vi "go.vi"(5 "dispense":T3={"Vacuum Setting (0000)"=0, "Pressure"=20, "on delay (ms)"=0.5, "off delay (ms) "=0.5} {"Vacuum Setting (0000)" min=0 max=1000 step=1 format="%04.0f"}, 7 "motion":T2, 8 "use new/data":bool, 9 "file path (dialog if empty)":path=path "D:/Gantry_General/Main/ms_kao/data/CAD PCB full 0.8 P30 20210608/CAD PCB full 0.8 P30 20210608.txt", 10 "cluster Array input":T5(array[cluster]), 11 "controller in":T4) -> (3 "controller out":T4)   [LabVIEW 2016]
uses:
  Classes/Controller/Motion/A3200 Folder/A3200.lvclass
  D:/Gantry_General/Classes/Controller/Motion/Motion Folder/Motion.lvclass
  Classes/Controller/Dispenser/Ultimus V2 Folder/Ultimus V2.lvclass
  Classes/Controller/I-O/NI-DAQ Folder/NI-DAQ.lvclass
  Classes/Controller/Motion/Motion Folder/Motion.lvclass
  Classes/Controller/I-O/I-O Folder/I-O.lvclass
  Classes/Controller/Dispenser/Dispenser Folder/Dispenser.lvclass
  <vilib>/Utility/file.llb/Read Delimited Spreadsheet (DBL).vi
  <vilib>/Utility/file.llb/Write Delimited Spreadsheet (I64).vi
panel:
  out "element":dbl
  out "all rows":dbl[][](array[numeric])
  out "draw point Cluster":T1
  out "Numeric":dbl=0.237
  out "i":i32=23
  out "size(s)":i32=75
  # "使用新/資料"
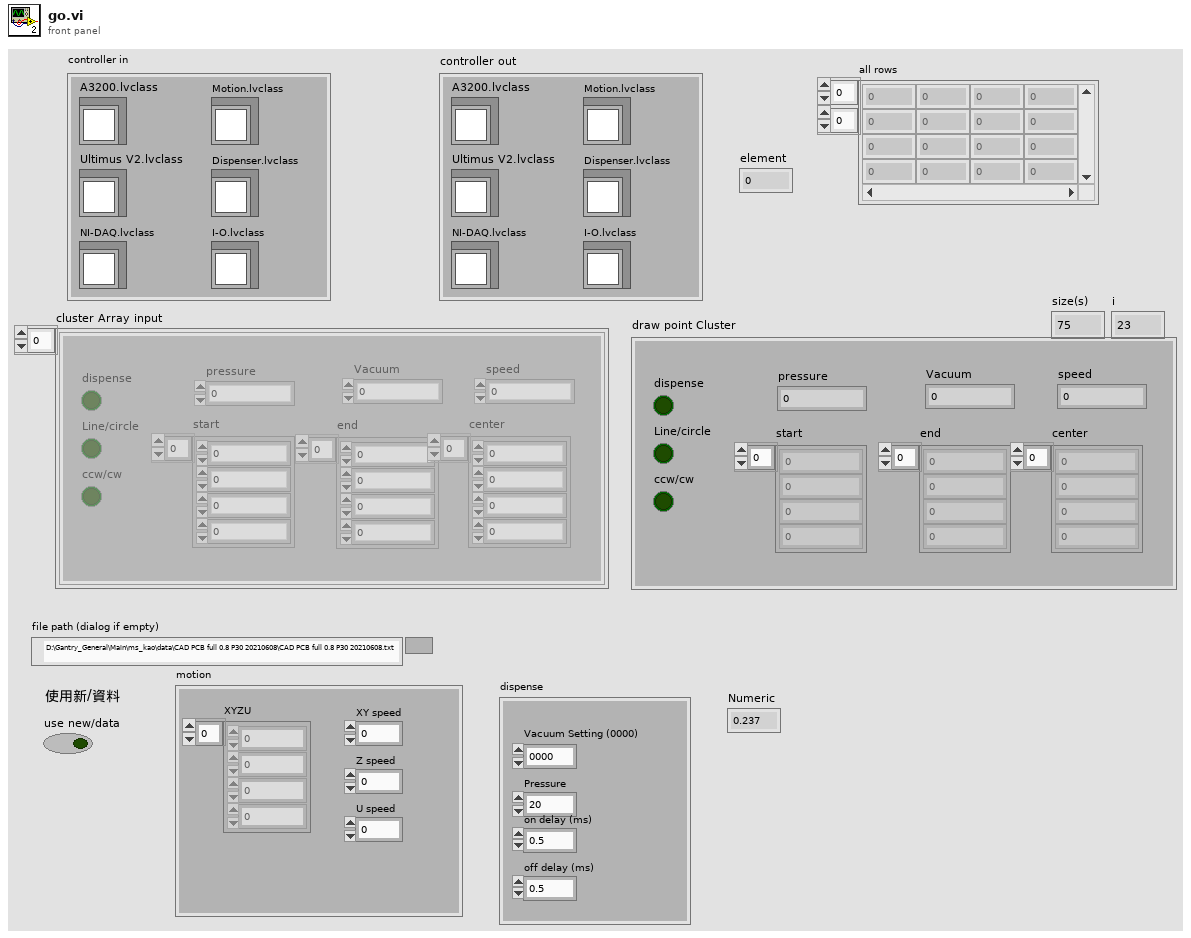
[diagram p1: front panel]
types:
  T1 = cluster{"dispense":bool, "Line/circle":bool, "ccw/cw":bool, "pressure":dbl, "speed":dbl, "start":dbl[], "end":dbl[], "center":dbl[], "Vacuum":dbl}
  T2 = cluster{"XYZU ":dbl[], "XY speed":dbl, "Z speed":dbl, "U speed":dbl}
  T3 = cluster{"Vacuum Setting (0000)":i64, "Pressure":i16, "on delay (ms)":dbl, "off delay (ms) ":dbl}
  T4 = cluster{"A3200.lvclass":refnum<class "A3200.lvclass">, "Ultimus V2.lvclass":refnum<class "Ultimus V2.lvclass">, "NI-DAQ.lvclass":refnum<class "NI-DAQ.lvclass">, "Motion.lvclass":refnum<class "Motion.lvclass">, "I-O.lvclass":refnum<class "I-O.lvclass">, "Dispenser.lvclass":refnum<class "Dispenser.lvclass">}
  T5 = cluster{"dispense":bool, "Line/circle":bool, "ccw/cw":bool, "pressure":dbl, "speed":dbl, "start":dbl[], "end":dbl[], "center":dbl[], "Vacuum":dbl}[]
  T6 = cluster{"file exists":bool, "dispense status now(on)":bool, "dispense status next(off)":bool, "dispense status IN":bool, "dispense status last":bool}
  T7 = typedef "dispense status data.ctl" = cluster{"file exists":bool, "dispense status now(on)":bool, "dispense status next(off)":bool, "dispense status IN":bool, "dispense status last":bool}
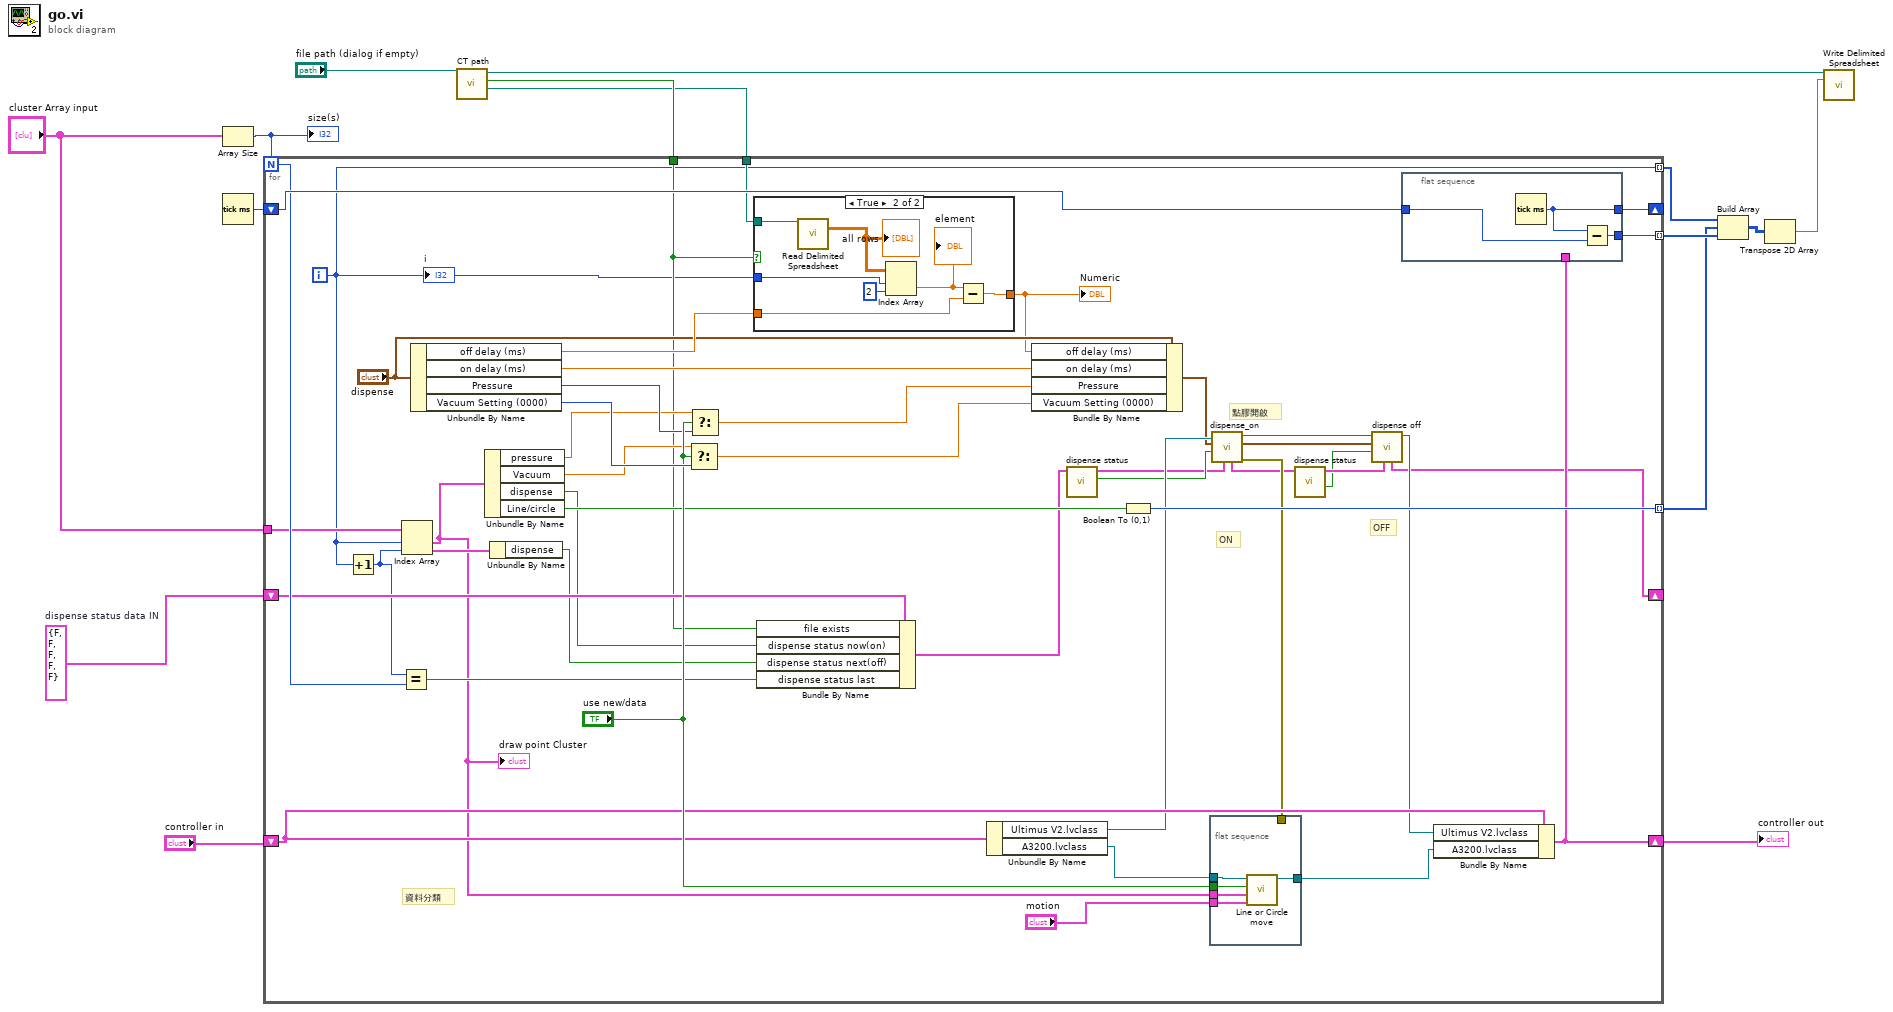
[diagram p0: block diagram]
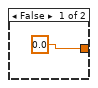
[diagram p2: hidden frame]
diagram:
  w1 = T6 {"file exists"=FALSE, "dispense status now(on)"=FALSE, "dispense status next(off)"=FALSE, "dispense status IN"=FALSE, "dispense status last"=FALSE}  # dispense status data IN
  n1 = Array Size(array="cluster Array input") -> (size(s)=w12:i32)
  "size(s)" <- w12
  n2 = Tick Count (ms)() -> (millisecond timer value=w11:u32)
  n3 = call "CT path.vi"("path"="file path (dialog if empty)") -> ("path 1"=w2:path, "file exists?"=w8:bool, "path 2"=w3:path)  [unwired: 8 in]
  n4 = for {
    N: w12 -> [w51]
    shift-right: [w60] -> _
    shift-left: w11 -> [w61]
    tunnel: [w59] -> w15 mode=indexing
    tunnel: [w58] -> w13 mode=indexing
    tunnel: "cluster Array input" -> [w28]
    tunnel: w8 -> [w29]
    tunnel: w2 -> [w57]
    tunnel: [w20] -> w6 mode=indexing
    shift-right: [w46] -> w4
    shift-left: "controller in" -> [w48]
    shift-right: [w24] -> _
    shift-left: w1 -> [w31]
    i -> [w20]
    # "OFF"
    # "ON"
    # "點膠開啟"
    # "資料分類"
    n5 = Increment(x=w20) -> (x+1=w27:i32)
    n6 = Equal?(x=w27, y=w51) -> (x = y?=w23:bool)
    n7 = Index Array(array=w28, index #1=w20, index #2=w27) -> (element #1=w16:T1, element #2=w26:T1)
    "draw point Cluster" <- w16
    n8 = Unbundle By Name("dispense") -> ("off delay (ms)"=w55:dbl, "on delay (ms)"=w41:dbl, "Pressure"=w49:i16, "Vacuum Setting (0000)"=w56:i64)
    n9 = Unbundle By Name(w16) -> ("pressure"=w37:dbl, "Vacuum"=w36:dbl, "dispense"=w21:bool, "Line/circle"=w50:bool)
    n10 = Unbundle By Name(w26) -> ("dispense"=w22:bool)
    n11 = Select(t=w36, s="use new/data", f=w56) -> (s? t:f=w38:dbl)
    n12 = Select(t=w37, s="use new/data", f=w49) -> (s? t:f=w39:dbl)
    n13 = case shown="True" w29 {
      tunnel: w57 -> [_ w74]
      tunnel: [0.0 ("f") w70] -> w40
      tunnel: w20 -> [_ w69]
      tunnel: w55 -> [_ w68]
      frame False {
      }
      frame True {
        n14 = call-poly <vilib>:"Read Delimited Spreadsheet.vi"("file path (dialog if empty)"=w74) -> ("all rows"=w72:dbl[][])  [unwired: 9 in, 5 out]
        "all rows" <- w72
        n15 = Index Array(array=w72, index (row)=w69, index (col)=2 ("disabled index (col)")) -> (element=w73:dbl)
        "element" <- w73
        n16 = Subtract(x=w73, y=w68) -> (x-y=w70:dbl)
      }
    }
    "Numeric" <- w40
    n17 = Bundle By Name(cluster=w31, "file exists"=w29, "dispense status now(on)"=w21, "dispense status next(off)"=w22, "dispense status last"=w23) -> (w30:T7)
    n18 = Unbundle By Name(w48) -> ("Ultimus V2.lvclass"=w45:refnum<class "Ultimus V2.lvclass">, "A3200.lvclass"=w52:refnum<class "A3200.lvclass">)
    n19 = Bundle By Name(cluster="dispense", "off delay (ms)"=w40, "on delay (ms)"=w41, "Pressure"=w39, "Vacuum Setting (0000)"=w38) -> (w43:T3)
    n20 = call "dispense status.vi"("dispense status data IN"=w30) -> ("dispense run on"=w32:bool, "dispense status data OUT"=w25:T7)  [unwired: 8 in, 1 out]
    n21 = Boolean To (0,1)(Boolean=w50) -> (0, 1=w58:i16)
    n22 = flat-sequence {
      tunnel: "use new/data" -> [w66]
      tunnel: w16 -> [w65]
      tunnel: "motion" -> [w64]
      tunnel: w44 -> [_]
      tunnel: [w63] -> w47
      tunnel: w52 -> [w62]
      frame #0 {
        n23 = call "Line or Circle move.vi"("motion"=w64, "draw point Cluster"=w65, "new/data speed"=w66, "Motion.lvclass"=w62) -> ("Motion.lvclass 2"=w63:refnum<class "A3200.lvclass">)  [unwired: 7 in]
      }
    }
    n24 = call "dispense_on.vi"("dispense status data IN"=w25, "dispense run on"=w32, "dispense in"=w43, "Ultimus V2.lvclass"=w45) -> ("error out"=w44:errorcluster, "dispense out"=w34:T3, "Ultimus V2.lvclass 2"=w33:refnum<class "Ultimus V2.lvclass">, "dispense status data OUT"=w19:T7)  [unwired: 4 in]
    n25 = call "dispense status.vi"("dispense status data IN"=w19) -> ("dispense run off"=w17:bool, "dispense status data OUT"=w18:T7)  [unwired: 8 in, 1 out]
    n26 = call "dispense off.vi"("dispense status data IN"=w18, "dispense run off"=w17, "dispense in"=w34, "Ultimus V2.lvclass"=w33) -> ("Ultimus V2.lvclass 2"=w35:refnum<class "Ultimus V2.lvclass">, "dispense status data OUT"=w24:T7)  [unwired: 4 in, 2 out]
    n27 = flat-sequence {
      tunnel: w61 -> [w77]
      tunnel: [w76] -> w60
      tunnel: [w75] -> w59
      tunnel: w46 -> [_]
      frame #0 {
        n28 = Tick Count (ms)() -> (millisecond timer value=w76:u32)
        n29 = Subtract(x=w76, y=w77) -> (x-y=w75:u32)
      }
    }
    n30 = Bundle By Name(cluster=w48, "Ultimus V2.lvclass"=w35, "A3200.lvclass"=w47) -> (w46:T4)
    "i" <- w20
  }
  "controller out" <- w4
  n31 = Build Array(w6, w13, w15) -> (w14:u32[][])
  n32 = Transpose 2D Array(2D array=w14) -> (transposed array=w7:u32[][])
  n33 = call-poly <vilib>:"Write Delimited Spreadsheet.vi"("file path (dialog if empty)"=w3, "2D data"=w7) -> ()  [unwired: 12 in, 2 out]
